vi "Read configuration.vi"(8 "error in":errorcluster, 11 "Benchmark PID editor node in":refnum<class "Benchmark PID editor node.lvclass">) -> (0 "error out":errorcluster, 2 "configuration":refnum<class "NISE_CEF_serializable configuration.lvclass">, 3 "Benchmark PID editor node out":refnum<class "Benchmark PID editor node.lvclass">)   [LabVIEW 2018, in "Benchmark PID editor node.lvclass"]
uses:
  Benchmark PID editor node.lvclass
  <vilib>/NI/Configuration Framework/serializable configuration/NISE_CEF_serializable configuration.lvclass
  Benchmark PID editor node.lvclass/Benchmark PID editor node.ctl
  module/configuration/Benchmark PID configuration.lvclass
  C:/Program Files (x86)/National Instruments/LabVIEW 2018/vi.lib/NI/Configuration Framework/serializable configuration/NISE_CEF_serializable configuration.lvclass
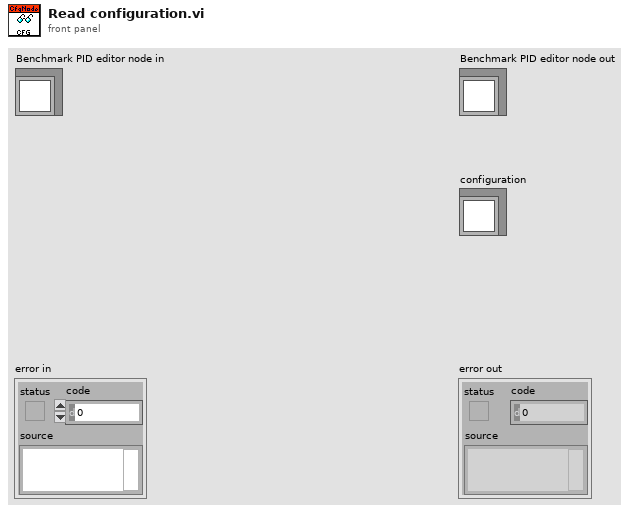
[diagram p1: front panel]
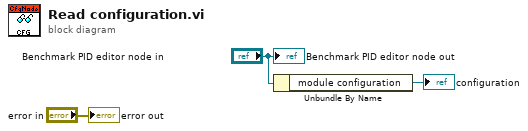
[diagram p0: block diagram]
diagram:
  n1 = Unbundle By Name("Benchmark PID editor node in") -> ("module configuration"=→"configuration":refnum<class "Benchmark PID configuration.lvclass">)
  "error out" <- "error in"
  "Benchmark PID editor node out" <- "Benchmark PID editor node in"
